vi "Calibrate_ESC.vi"(1 "Calibrate?":bool, 2 "PWM Frequency":dbl=50.0 format="%#_13g", 3 "Min Duty Cycle (%)":dbl=5.0 format="%#_13g", 4 "Max Duty Cycle (%)":dbl=10.0 format="%#_13g") -> ()   [LabVIEW 2015]
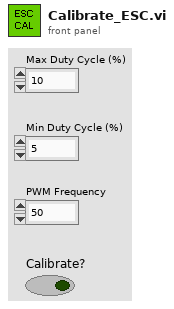
[diagram p1: front panel]
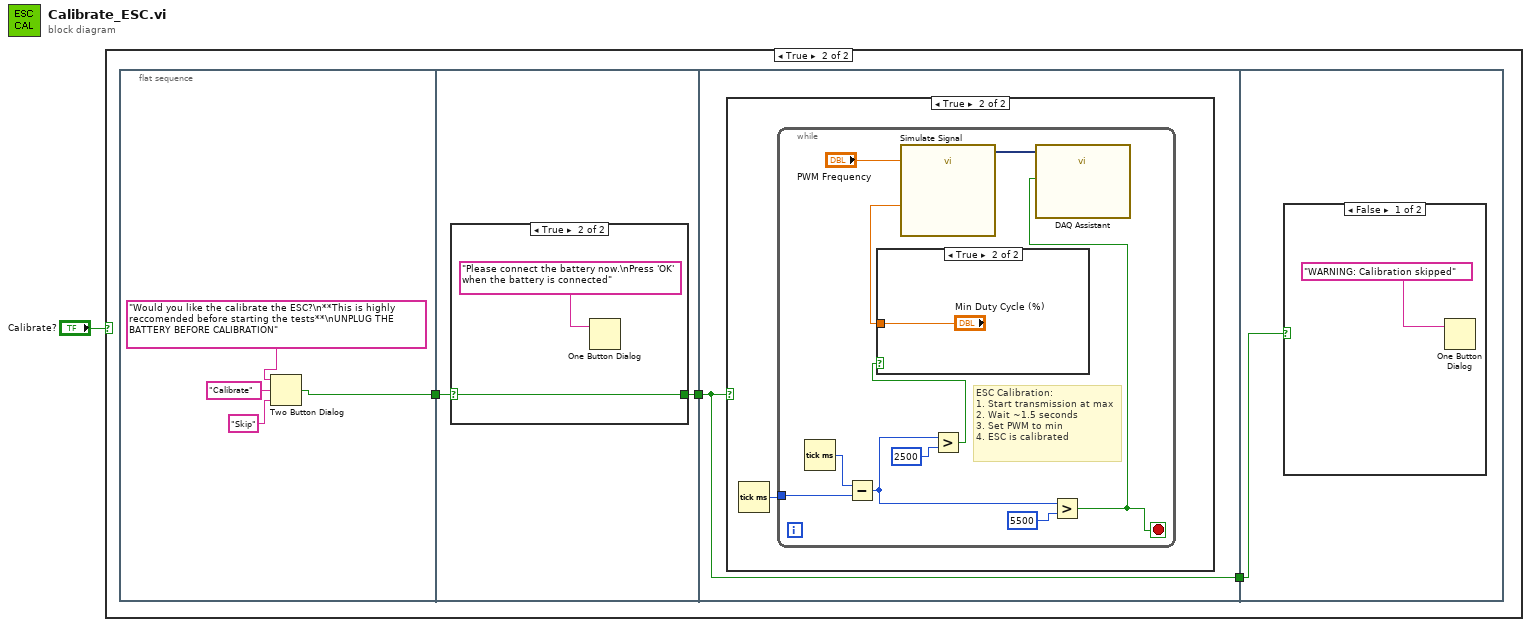
[diagram p0: block diagram]
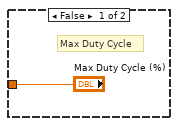
[diagram p5: hidden frame]
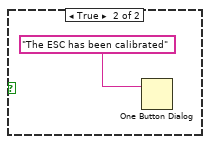
[diagram p6: hidden frame]
diagram:
  n1 = case shown="True" "Calibrate?" {
    frame False {
    }
    frame True {
      n2 = flat-sequence {
        tunnel: [w5] -> w4
        tunnel: w4 -> [w10]
        tunnel: [w9] -> w3
        tunnel: w3 -> [w14]
        tunnel: [w14] -> w2
        tunnel: w2 -> [w28]
        frame #0 {
          n3 = Two Button Dialog(message="Would you like the calibrate the ESC?\n**This is highly reccomended before starting the tests**\nUNPLUG THE BATTERY BEFORE CALIBRATION", 1:"Skip" ("F button name (\"Cancel\")"), 2:"Calibrate" ("T button name (\"OK\")")) -> (T button?=w5:bool)
        }
        frame #1 {
          n4 = case shown="True" w10 {
            selector: w10 -> [w11 w13]
            tunnel: [w11 w13] -> w9
            frame False {
            }
            frame True {
              n5 = One Button Dialog(message="Please connect the battery now.\nPress 'OK' when the battery is connected") -> ()  [unwired: 1 in, 1 out]
            }
          }
        }
        frame #2 {
          n6 = case shown="True" w14 {
            frame False {
              # "Do not Calibrate if false."
            }
            frame True {
              n7 = Tick Count (ms)() -> (millisecond timer value=w15:u32)
              n8 = while {
                tunnel: w15 -> [w24]
                stop <- w17 stop-if-true
                # "ESC Calibration:\n1. Start transmission at max\n2. Wait ~1.5 seconds\n3. Set PWM to min\n4. ESC is calibrated"
                n9 = Tick Count (ms)() -> (millisecond timer value=w22:u32)
                n10 = Subtract(x=w22, y=w24) -> (x-y=w19:u32)
                n11 = Greater?(x=w19, y=u32 2500) -> (0:w20:bool)
                n12 = case shown="True" w20 {
                  tunnel: ["Max Duty Cycle (%)" "Min Duty Cycle (%)"] -> w21
                  frame False {
                    # "Max Duty Cycle"
                  }
                  frame True {
                  }
                }
                n13 = call "Simulate Signal"("Duty Cycle (%)"=w21, "Frequency"="PWM Frequency") -> ("Square"=w25:dynamicdata)  [unwired: 12 in, 1 out]
                n14 = Greater?(x=w19, y=u32 5500) -> (0:w17:bool)
                n15 = call "DAQ Assistant"("data"=w25, "stop (F)"=w17) -> ()  [unwired: 15 in, 3 out]
              }
            }
          }
        }
        frame #3 {
          n16 = case shown="False" w28 {
            frame False {
              n17 = One Button Dialog(message="WARNING: Calibration skipped") -> ()  [unwired: 1 in, 1 out]
            }
            frame True {
              n18 = One Button Dialog(message="The ESC has been calibrated") -> ()  [unwired: 1 in, 1 out]
            }
          }
        }
      }
    }
  }
